vi "总处理函数.vi"(8 "error in":errorcluster, 9 "Image IN 2":T1(plugin-control), 11 "Image IN":T1(plugin-control)) -> (0 "error out":errorcluster, 1 "Image O1":T1(plugin-control), 3 "Image O2":T1(plugin-control))   [LabVIEW 2017]
uses:
  Global System.vi
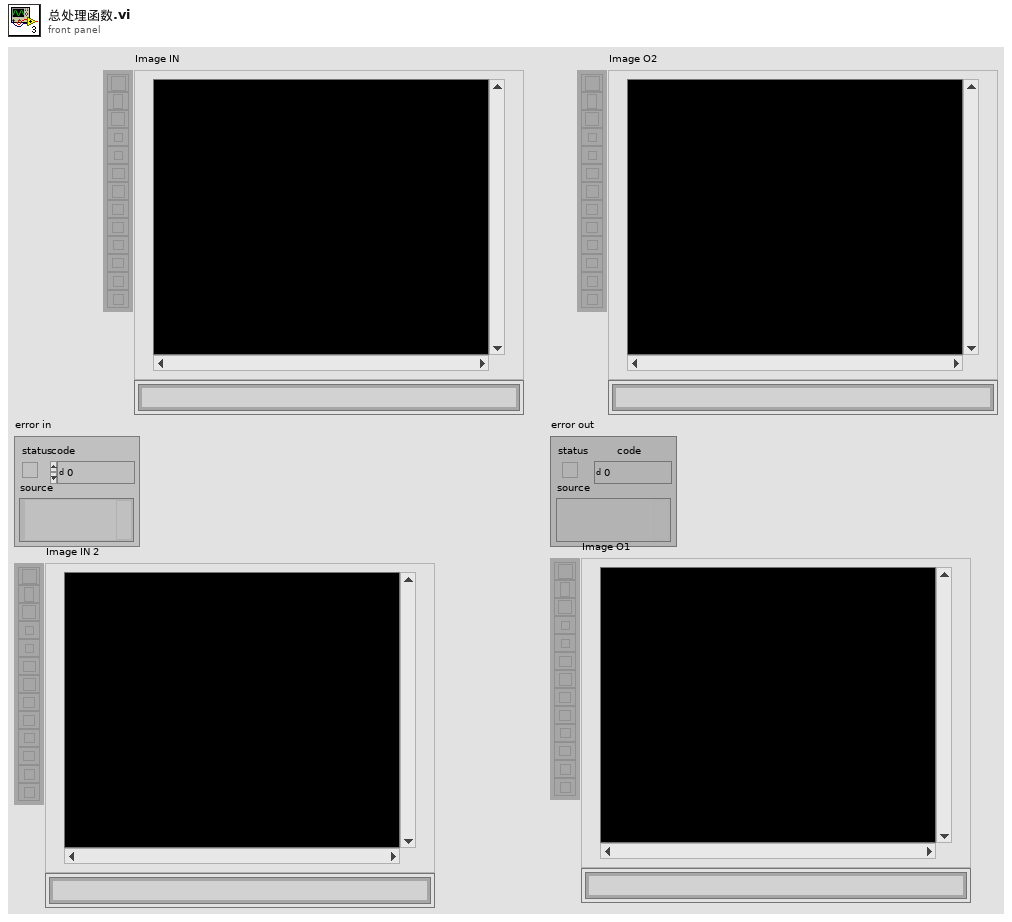
[diagram p1: front panel]
types:
  T1 = typedef "IMAQ Image.ctl" = refnum<image>
  T2 = cluster{"扇区个数":string, "Fitted Circle (Find Circular Edge 1)":cluster{"Center (Pixels)":cluster{"X":sgl, "Y":sgl}, "Radius (Pixels)":dbl, "Center (Real-World)":cluster{"X":sgl, "Y":sgl}, "Radius (Real-World)":dbl, "Roundness (Real-World)":dbl, "Average Strength":dbl, "Average SNR (dB)":dbl}, "Range (Threshold 1)":cluster{"Lower value":sgl, "Upper value":sgl}, "Process (Edge Detector 1)":enum16{"Get First Edge", "Get First + Last Edge", "Get All Edges", "Get Best Edge"}, "Edge Options (Edge Detector 1)":cluster{"Edge Polarity":u32, "Kernel Size":u32, "Width":u32, "Minimum Edge Strength":sgl, "Interpolation Type":enum32{"Zero Order", "Bilinear", "Quadratic", "Cubic", "Bilinear Fixed"}, "Data Processing Method":enum32{"Average", "Median"}}}
  T3 = typedef "ROI Descriptor" = cluster{"Global Rectangle":i32[], "Contours":cluster{"ID":enum32{"External", "Internal"}, "Type":u32, "Coordinates":i32[]}[]}
  T4 = typedef "Edge Options.ctl" = cluster{"Edge Polarity":T5, "Kernel Size":u32, "Width":u32, "Minimum Edge Strength":sgl, "Interpolation Type":enum32{"Zero Order", "Bilinear", "Quadratic", "Cubic", "Bilinear Fixed"}, "Data Processing Method":enum32{"Average", "Median"}}
  T5 = typedef "Edge Polarity.ctl" = u32
  T6 = cluster{"Search  Direction":u32, "Edge Options":T4, "Show Search Area":bool, "Show Search Lines":bool, "Show Edges Found":bool, "Show Result":bool, "Search Area Color":u32, "Search Lines Color":u32, "Edge Locations Color":u32, "Result Color":u32, "Overlay Group Name":string}
  T7 = cluster{"Center (Pixels)":cluster{"X":sgl, "Y":sgl}, "Radius (Pixels)":dbl, "Center (Real-World)":cluster{"X":sgl, "Y":sgl}, "Radius (Real-World)":dbl, "Roundness (Real-World)":dbl, "Average Strength":dbl, "Average SNR (dB)":dbl}
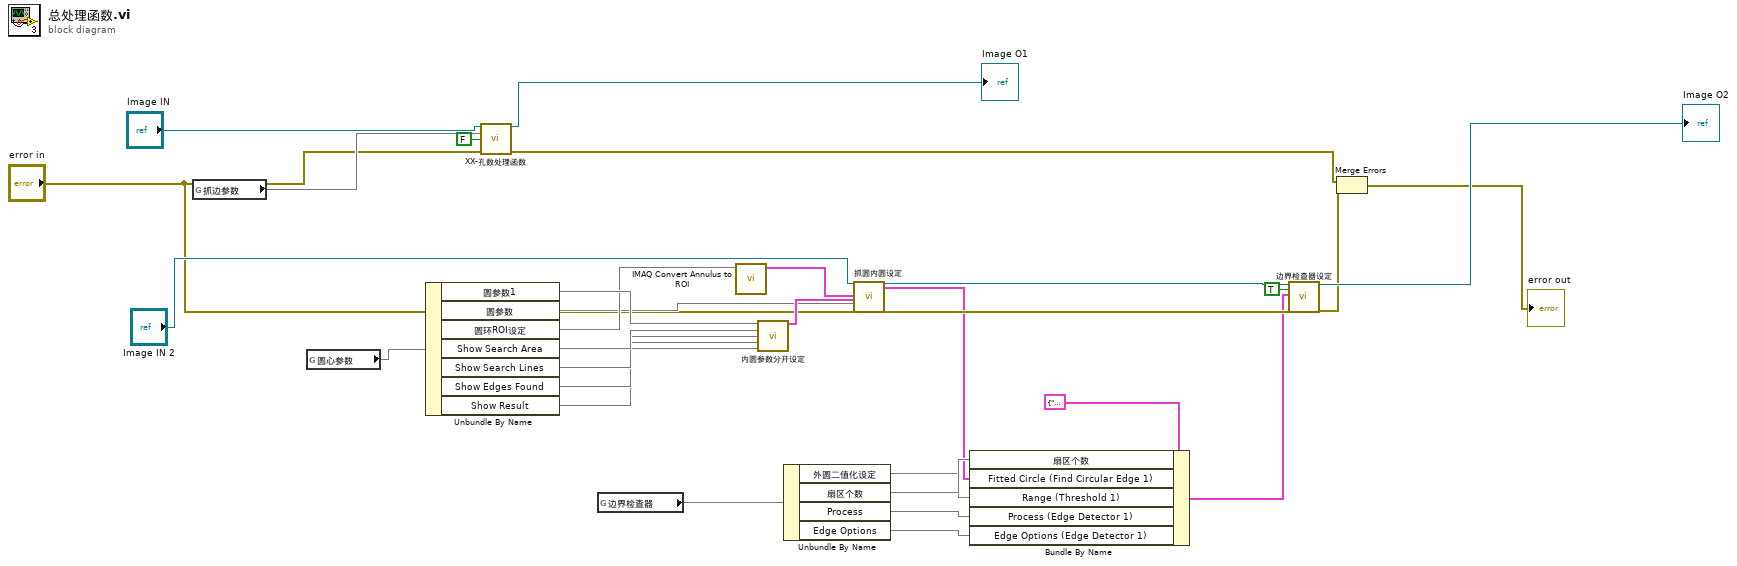
[diagram p0: block diagram]
diagram:
  n1 = global read "Global System.vi" "抓边参数"() -> (w30)
  n2 = global read "Global System.vi" "圆心参数"() -> (w24)
  n3 = Unbundle By Name(w24) -> ("圆参数1"=w23, "圆参数"=w16, "圆环ROI设定"=w18, "Show Search Area"=w22, "Show Search Lines"=w21, "Show Edges Found"=w20, "Show Result"=w19)
  n4 = call "XX-孔数处理函数.vi"("Image in"="Image IN", "参数输入"=w30, "图像处理开关"=FALSE, "error in"="error in") -> ("Image Out"=→"Image O1":T1, "error out"=w5:errorcluster)  [unwired: 9 in, 1 out]
  n5 = global read "Global System.vi" "边界检查器"() -> (w11)
  n6 = call "IMAQ Convert Annulus to ROI"("Annulus"=w18) -> ("ROI Descriptor"=w28:T3)  [unwired: 8 in, 1 out]
  n7 = call "内圆参数分开设定.vi"("内圆参数in"=w23, "Show Search Area"=w22, "Show Search Lines"=w21, "Show Edges Found"=w20, "Show Result"=w19) -> ("our"=w29:T6)  [unwired: 10 in]
  n8 = Unbundle By Name(w11) -> ("外圆二值化设定"=w12, "扇区个数"=w15, "Process"=w14, "Edge Options"=w13)
  n9 = call "抓圆内圆设定"("Image In"="Image IN 2", "ROI Descriptor (Find Circular Edge 1)"=w28, "Options (Find Circular Edge 1)"=w29, "Circle Fit Options (Find Circular Edge 1)"=w16, "error in"="error in") -> ("Image Out"=w27:T1, "Fitted Circle (Find Circular Edge 1)"=w10:T7, "error out"=w25:errorcluster)  [unwired: 20 in]
  n10 = Bundle By Name(cluster=T2 {"扇区个数"="1", "Fitted Circle (Find Circular Edge 1)"={"Center (Pixels)"={"X"=1736.0, "Y"=1501.0}, "Radius (Pixels)"=1442.0, "Center (Real-World)"={"X"=1736.0, "Y"=1501.0}, "Radius (Real-World)"=1442.0, "Roundness (Real-World)"=0.0, "Average Strength"=0.0, "Average SNR (dB)"=0.0}, "Range (Threshold 1)"={"Lower value"=65.0, "Upper value"=255.0}, "Process (Edge Detector 1)"=enum."Get All Edges", "Edge Options (Edge Detector 1)"={"Edge Polarity"=0, "Kernel Size"=9, "Width"=5, "Minimum Edge Strength"=27.0, "Interpolation Type"=enum."Bilinear", "Data Processing Method"=enum."Average"}} ("边界检查器参数"), "扇区个数"=w15, "Fitted Circle (Find Circular Edge 1)"=w10, "Range (Threshold 1)"=w12, "Process (Edge Detector 1)"=w14, "Edge Options (Edge Detector 1)"=w13) -> (w8:T2)
  n11 = call "边界检查器设定.vi"("Image IN"=w27, "启动变量"=TRUE, "边界检查器参数"=w8, "error in"=w25) -> ("Image Out"=→"Image O2":T1, "error out"=w4:errorcluster)  [unwired: 11 in, 3 out]
  n12 = Merge Errors(w5, w4) -> (→"error out":errorcluster)
